vi "Read YB.vi"(11 "HE_state in":refnum<class "HE_state.lvclass">) -> (2 "YB":bool[](array[boolean]), 3 "HE_state out":refnum<class "HE_state.lvclass">)   [LabVIEW 2019, in "Heating.lvlib" / "HE_state.lvclass"]
uses:
  HE_state.lvclass
  HE_state.lvclass/HE_state.ctl
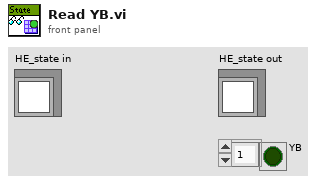
[diagram p1: front panel]
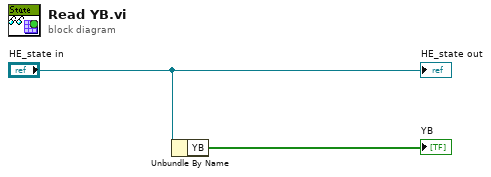
[diagram p0: block diagram]
diagram:
  n1 = Unbundle By Name("HE_state in") -> ("YB"=→"YB":bool[])
  "HE_state out" <- "HE_state in"
